vi "Correct_Position_info_NM2.vi"() -> (0 "error out":errorcluster)   [LabVIEW 2011]
panel:
  in  "Folder of RD Folders":path
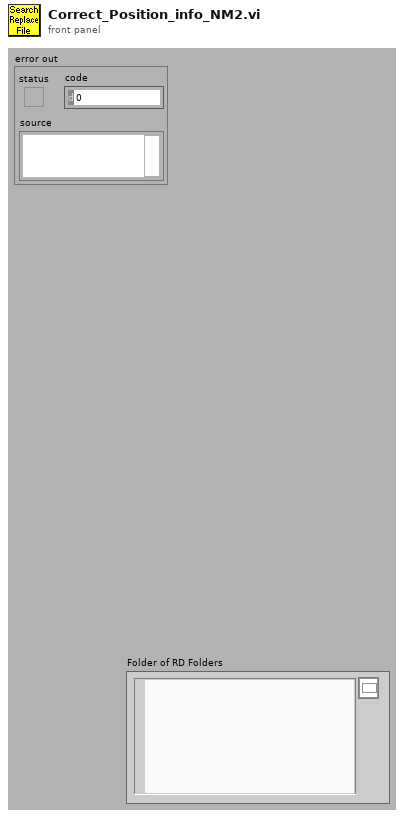
[diagram p1: front panel]
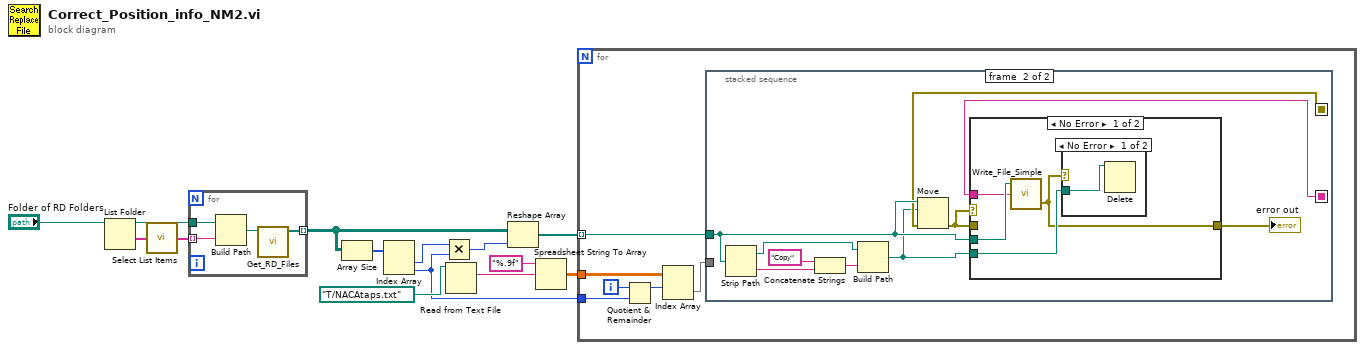
[diagram p0: block diagram]
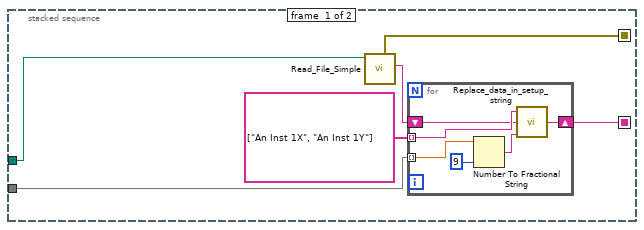
[diagram p2: hidden frame]
diagram:
  n1 = List Folder(path="Folder of RD Folders") -> (path out=w8:path, folder names=w9:string[])  [unwired: 3 in, 2 out]
  n2 = call "Select List Items.vi"("Item Names"=w9) -> ("Selected Items"=w7:string[])  [unwired: 4 in]
  n3 = for {
    tunnel: w8 -> [w17]
    tunnel: w7 -> [w16] mode=indexing
    tunnel: [w15] -> w3 mode=indexing
    n4 = Build Path(base path=w17, name or relative path=w16) -> (appended path=w18:path)
    n5 = call "Get_RD_Files.vi"("Raw Data File Folder"=w18) -> ("Array of only RD Files"=w15:path[])  [unwired: 10 in]
  }
  n6 = Array Size(array=w3) -> (size(s)=w4:i32[])
  n7 = Index Array(array=w4) -> (element #1=w5:i32, element #2=w1:i32)  [unwired: 2 in]
  n8 = Multiply(x=w5, y=w1) -> (x*y=w6:i32)
  n9 = Read from Text File(file (use dialog)=path "T:/NACAtaps.txt") -> (text=w13:string)  [unwired: 3 in, 3 out]
  n10 = Reshape Array(w3, w6) -> (w2:path[])
  n11 = Spreadsheet String To Array(format string="%.9f", spreadsheet string=w13) -> (array=w11:dbl[][])  [unwired: 2 in]
  n12 = for {
    tunnel: w2 -> [w22] mode=indexing
    tunnel: w11 -> [w24]
    tunnel: w1 -> [w20]
    i -> [w21]
    n13 = Quotient & Remainder(x=w21, y=w20) -> (x-y*floor(x/y)=w19:i32)  [unwired: 1 out]
    n14 = Index Array(array=w24, index (row)=w19) -> (element=w23:dbl[])  [unwired: 1 in]
    n15 = stacked-sequence {
      seq-local: [w30 _] -> [_ w43]
      seq-local: [w28 _] -> [_ w44]
      tunnel: w22 -> [w26 w46]
      tunnel: w23 -> [w25 _]
      frame #0 {
        n16 = call "Read_File_Simple.vi"("Filename"=w26) -> ("error out"=w30:errorcluster, "string"=w27:string)  [unwired: 4 in, 4 out]
        n17 = for {
          shift-right: [w34] -> w28
          shift-left: w27 -> [w35]
          tunnel: string[] ["An Inst 1X", "An Inst 1Y"] -> [w36] mode=indexing
          tunnel: w25 -> [w31] mode=indexing
          n18 = Number To Fractional String(number=w31, precision (6)=i16 9) -> (F-format string=w32:string)  [unwired: 2 in]
          n19 = call "Replace_data_in_setup_string.vi"("New data string"=w32, "Input string"=w35, "Variable name"=w36) -> ("Appended string"=w34:string)
        }
      }
      frame #1 {
        n20 = Strip Path(path=w46) -> (stripped path=w39:path, name=w41:string)
        n21 = Concatenate Strings("Copy" ("name or relative path"), w41) -> (w40:string)
        n22 = Build Path(base path=w39, name or relative path=w40) -> (appended path=w38:path)
        n23 = Move(source path=w46, error in=w43, 10:w38) -> (error out=w37:errorcluster)  [unwired: 2 in, 2 out]
        n24 = case shown="No Error" w37 {
          tunnel: w46 -> [w50 _]
          tunnel: w44 -> [w49 _]
          tunnel: w38 -> [w48 _]
          tunnel: [w47 w52] -> w45
          tunnel: w37 -> [_ w52]
          frame No Error {
            n25 = call "Write_File_Simple.vi"("character string"=w49, "file path"=w50) -> ("error out"=w47:errorcluster)  [unwired: 1 in, 1 out]
            n26 = case shown="No Error" w47 {
              tunnel: w48 -> [w51 _]
              frame No Error {
                n27 = Delete(path (use dialog)=w51) -> ()  [unwired: 4 in, 3 out]
              }
              frame Error {
              }
            }
          }
          frame Error {
          }
        }
        "error out" <- w45
      }
    }
  }
